vi "MFC Init.vi"(8 "error in (no error)":errorcluster, 11 "Cluster in":T2) -> (0 "error out":errorcluster, 1 "MFC Range":i32, 2 "Disabled":T3(ring), 3 "Cluster out":T2)   [LabVIEW 2015]
panel:
  out "substring before match":string
  out "MFC Info":T1
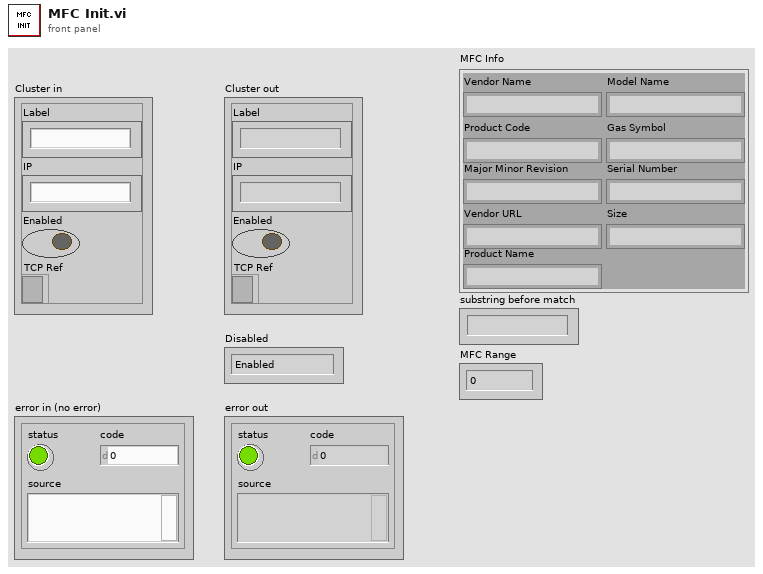
[diagram p1: front panel]
types:
  T1 = cluster{"Vendor Name":string, "Product Code":string, "Major Minor Revision":string, "Vendor URL":string, "Product Name":string, "Model Name":string, "Gas Symbol":string, "Serial Number":string, "Size":string}
  T2 = cluster{"Label":string, "IP":string, "Enabled":bool, "TCP Ref":refnum<k5>}
  T3 = enum8{"Enabled", "Disabled", "Disabled and Grayed Out"}
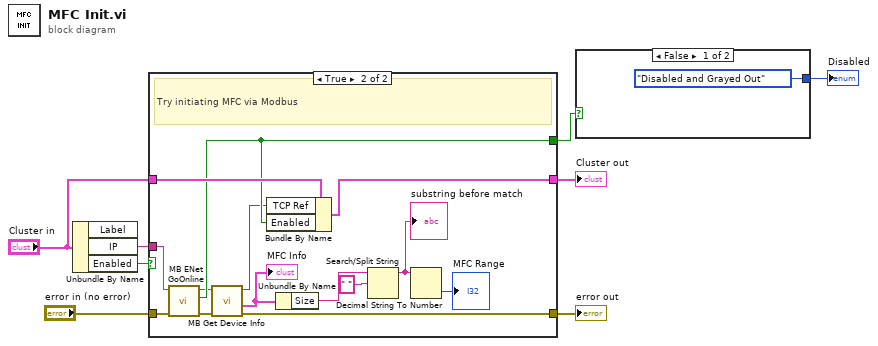
[diagram p0: block diagram]
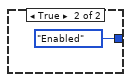
[diagram p2: hidden frame]
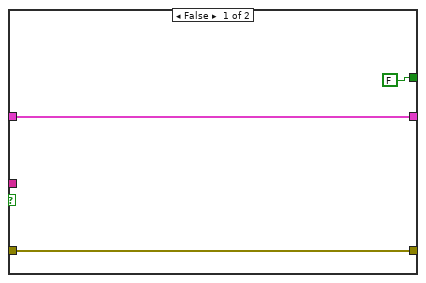
[diagram p3: hidden frame]
diagram:
  n1 = Unbundle By Name("Cluster in") -> ("IP"=w1:string, "Enabled"=w5:bool)  [unwired: 1 out]
  n2 = case shown="True" w5 {
    tunnel: "error in (no error)" -> [w11 w25]
    tunnel: [w11 w18] -> w7
    tunnel: w1 -> [_ w24]
    tunnel: "Cluster in" -> [w10 w23]
    tunnel: [w10 w22] -> w4
    tunnel: [FALSE ("OK") w21] -> w8
    frame False {
    }
    frame True {
      # "Try initiating MFC via Modbus"
      n3 = call "MB ENet GoOnline.vi"("error in (no error)"=w25, "IP Address"=w24) -> ("error out"=w19:errorcluster, "OK"=w21:bool, "TCP Ref"=w20:refnum<k5>)  [unwired: 7 in]
      n4 = call "MB Get Device Info.vi"("error in (no error)"=w19, "TCP Ref:ValBlock"=w20) -> ("error out"=w18:errorcluster, "MFC Info"=w16:T1, "dup TCP Ref:ValBlock"=w17:refnum<k5>)  [unwired: 7 in]
      "MFC Info" <- w16
      n5 = Bundle By Name(cluster=w23, "TCP Ref"=w17, "Enabled"=w21) -> (w22:T2)
      n6 = Unbundle By Name(w16) -> ("Size"=w15:string)
      n7 = Search/Split String(string=w15, search string/char (-)=" ") -> (substring before match=w13:string)  [unwired: 1 in, 2 out]
      "substring before match" <- w13
      n8 = Decimal String To Number(string=w13) -> (number=→"MFC Range":i32)  [unwired: 2 in, 1 out]
    }
  }
  "error out" <- w7
  "Cluster out" <- w4
  n9 = case shown="False" w8 {
    tunnel: [T3."Disabled and Grayed Out" ("Disabled") T3."Enabled" ("Disabled")] -> w6
    frame False {
    }
    frame True {
    }
  }
  "Disabled" <- w6
